vi "Write Data to File.vi"(8 "error in (no error)":errorcluster, 10 "data":waveform(dbl)[](array[waveform]), 11 "Logger in":refnum<class "Logger.lvclass">) -> (0 "error out":errorcluster, 3 "Logger out":refnum<class "Logger.lvclass">)   [LabVIEW 2026, in "Logger.lvlib" / "Logger.lvclass"]
uses:
  Logger.lvclass
  C:/Program Files/National Instruments/LabVIEW 2026/vi.lib/ActorFramework/Actor/Actor.lvclass
  Logger.lvclass/Logger.ctl
  <vilib>/ActorFramework/Actor/Actor.lvclass/Actor.ctl
  <vilib>/ActorFramework/Message Enqueuer/Message Enqueuer.lvclass/Message Enqueuer.ctl
  config/Logger Configuration.lvclass/Logger Configuration.ctl
  Logger Messages/Send File to Server Msg/Send File to Server Msg.lvclass/Send File to Server Msg.ctl
  config/Read Logging Settings.vi
  <vilib>/ActorFramework/Message Enqueuer/Init from Existing Queue.vi
  <vilib>/ActorFramework/Message Enqueuer/Enqueue.vi
  Logger Messages/Send File to Server Msg/Send File to Server Msg.lvclass
  C:/Program Files/National Instruments/LabVIEW 2026/vi.lib/ActorFramework/Message/Message.lvclass
  <vilib>/ActorFramework/Message Priority Queue/Priority Enqueue.vi
  <vilib>/ActorFramework/Message Enqueuer/Message Enqueuer.lvclass
  <vilib>/ActorFramework/Actor/Actor.lvclass
  config/Logger Configuration.lvclass
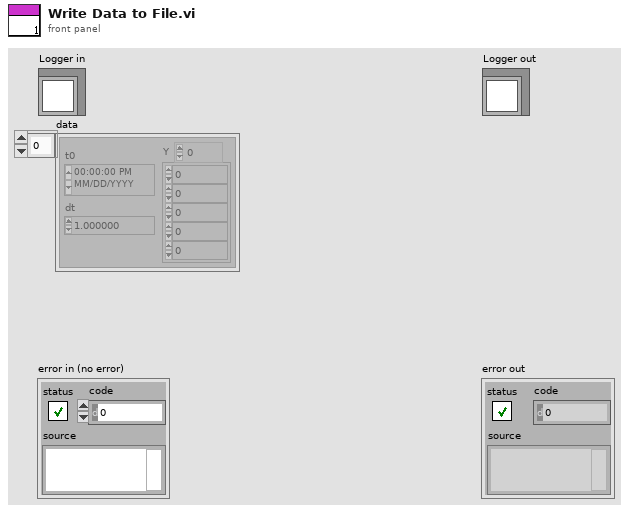
[diagram p1: front panel]
types:
  T1 = cluster{"File Name":string, "Upload Files to SystemLink Server":bool, "Max Samples Per File":i32, "Folder Location":path, "Logging":bool}
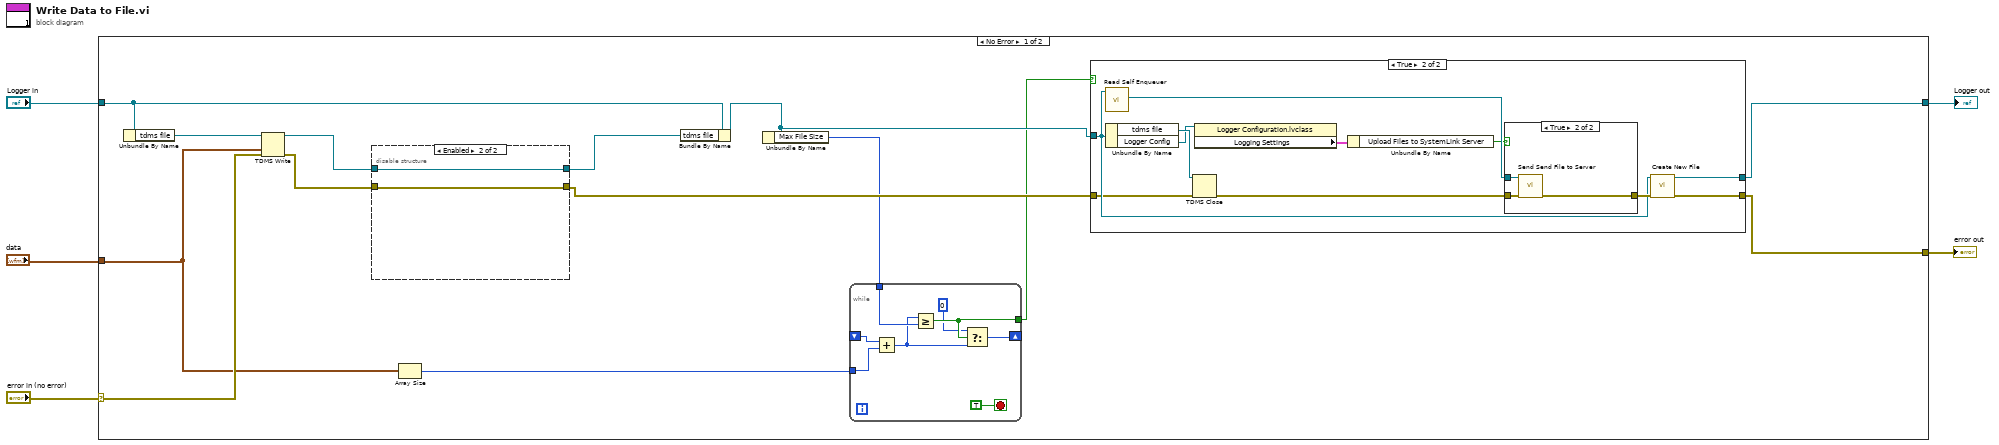
[diagram p0: block diagram]
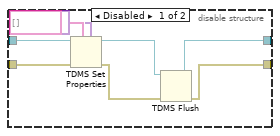
[diagram p4: hidden frame]
diagram:
  n1 = case shown="No Error" "error in (no error)" {
    selector: "error in (no error)" -> [w17 w56]
    tunnel: [w13 w56] -> w4
    tunnel: [w14 w55] -> w2
    tunnel: "Logger in" -> [w19 w55]
    tunnel: "data" -> [w10 _]
    frame No Error {
      n2 = Unbundle By Name(w19) -> ("tdms file"=w18:refnum<k34>)
      n3 = TDMS Write(0:w18, 9:w10, 11:w17) -> (4:w16:refnum<k34>, 15:w15:errorcluster)  [unwired: 3 in, 2 out]
      n4 = disable-structure shown="Enabled" {
        disable-tunnel: w16 -> [w52 w54]
        disable-tunnel: [w47 w54] -> w11
        disable-tunnel: w15 -> [w50 w53]
        disable-tunnel: [w48 w53] -> w12
        frame Disabled {
          n5 = TDMS Set Properties(5:variant[] [] ("property values"), 7:string[] [] ("property names"), 8:w50, 11:w52) -> (0:w49:errorcluster, 3:w51:refnum<k34>)  [unwired: 2 in, 2 out]
          n6 = TDMS Flush(4:w49, 7:w51) -> (0:w48:errorcluster, 3:w47:refnum<k34>)
        }
        frame Enabled {
        }
      }
      n7 = Array Size(array=w10) -> (size(s)=w9:i32)
      n8 = Bundle By Name(cluster=w19, "tdms file"=w11) -> (w8:refnum<class "Logger.lvclass">)
      n9 = Unbundle By Name(w8) -> ("Max File Size"=w7:i32)
      n10 = while {
        tunnel: w9 -> [w27]
        shift-right: [w21] -> _
        shift-left: _ -> [w26]
        tunnel: w7 -> [w24]
        tunnel: [w23] -> w6
        stop <- TRUE stop-if-true
        n11 = Add(x=w26, y=w27) -> (x+y=w22:i32)
        n12 = Greater Or Equal?(x=w22, y=w24) -> (x >= y?=w23:bool)
        n13 = Select(t=0, s=w23, f=w22) -> (s? t:f=w21:i32)
      }
      n14 = case shown="True" w6 {
        tunnel: w8 -> [w29 w36]
        tunnel: [w29 w40] -> w14
        tunnel: w12 -> [w28 w34]
        tunnel: [w28 w39] -> w13
        frame False {
        }
        frame True {
          n15 = call <vilib>:"Read Self Enqueuer.vi"("Actor"=w36) -> ("Self Enqueuer"=w38:refnum<class "Message Enqueuer.lvclass">)  [unwired: 10 in]
          n16 = Unbundle By Name(w36) -> ("tdms file"=w35:refnum<k34>, "Logger Config"=w32:refnum<class "Logger Configuration.lvclass">)
          n17 = TDMS Close(8:w34, 11:w35) -> (0:w33:errorcluster)  [unwired: 1 out]
          n18 = property class="Logger Configuration.lvclass"(reference=w32) -> ("Logging Settings"=w31:T1)  [unwired: 1 in, 2 out]
          n19 = Unbundle By Name(w31) -> ("Upload Files to SystemLink Server"=w30:bool)
          n20 = case shown="True" w30 {
            tunnel: w38 -> [_ w44]
            tunnel: [w41 w43] -> w37
            tunnel: w33 -> [w41 w42]
            frame False {
            }
            frame True {
              n21 = call "Send Send File to Server.vi"("error in (no error)"=w42, "Message Enqueuer"=w44) -> ("error out"=w43:errorcluster)  [unwired: 8 in, 1 out]
            }
          }
          n22 = call-dynamic "Create New File.vi"("error in (no error)"=w37, "Logger in"=w36) -> ("error out"=w39:errorcluster, "Logger out"=w40:refnum<class "Logger.lvclass">)  [unwired: 8 in]
        }
      }
    }
    frame Error {
    }
  }
  "error out" <- w4
  "Logger out" <- w2
